vi "历史记录.vi"(9 "动作":enum16{"读取", "添加", "删除", "初始化"}(ring), 11 "历史曲线":cluster{"时间":dbl[], "力":dbl[]}[](array[cluster])) -> (0 "错误输出":errorcluster, 1 "记录大小":i32, 3 "历史曲线":cluster{"时间":dbl[], "力":dbl[]}[](array[cluster]))   [LabVIEW 2015]
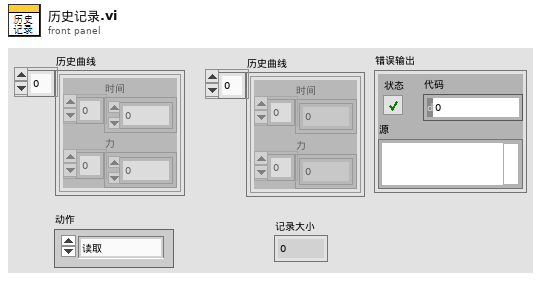
[diagram p1: front panel]
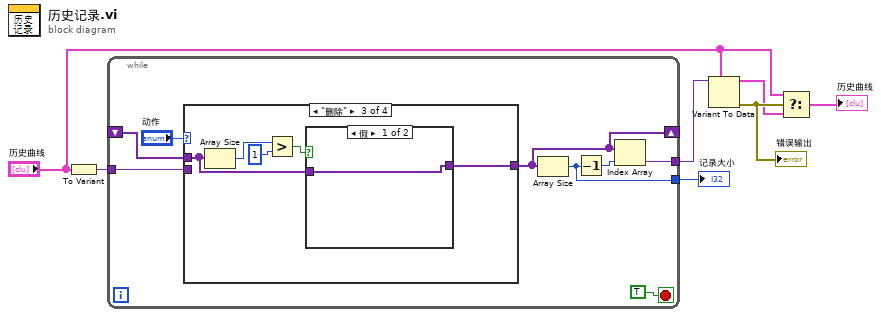
[diagram p0: block diagram]
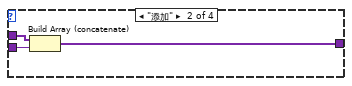
[diagram p3: hidden frame]
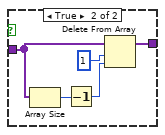
[diagram p4: hidden frame]
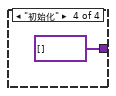
[diagram p5: hidden frame]
diagram:
  n1 = To Variant(anything="历史曲线") -> (Variant=w7:variant)
  n2 = while {
    shift-right: [w8] -> _
    shift-left: _ -> [w13]
    tunnel: w7 -> [w14]
    tunnel: [w11] -> w6
    tunnel: [w9] -> w5
    stop <- TRUE stop-if-true
    n3 = case shown="\"删除\"" "动作" {
      tunnel: w14 -> [_ w18 _ _]
      tunnel: [w16 w17 w24 variant[] []] -> w8
      tunnel: w13 -> [w16 w19 w23 _]
      frame "读取", Default {
      }
      frame "添加" {
        n4 = Build Array (concatenate)(w19, w18) -> (w17:variant[])
      }
      frame "删除" {
        n5 = Array Size(array=w23) -> (size(s)=w22:i32)
        n6 = Greater?(x=w22, y=1) -> (0:w20:bool)
        n7 = case shown="假" w20 {
          tunnel: [w25 w28] -> w24
          tunnel: w23 -> [w25 w26]
          frame False {
          }
          frame True {
            n8 = Array Size(array=w26) -> (size(s)=w29:i32)
            n9 = Decrement(x=w29) -> (x-1=w27:i32)
            n10 = Delete From Array(array=w26, length=1 ("长度"), index=w27) -> (array with subset deleted=w28:variant[])  [unwired: 1 out]
          }
        }
      }
      frame "初始化" {
      }
    }
    n11 = Array Size(array=w8) -> (size(s)=w9:i32)
    n12 = Decrement(x=w9) -> (x-1=w10:i32)
    n13 = Index Array(array=w8, index=w10) -> (element=w11:variant)
  }
  "记录大小" <- w5
  n14 = Variant To Data(type="历史曲线", Variant=w6) -> (data=w3:cluster{"时间":dbl[], "力":dbl[]}[], error out=w4:errorcluster)  [unwired: 1 in]
  "错误输出" <- w4
  n15 = Select(t="历史曲线", s=w4, f=w3) -> (s? t:f=→"历史曲线":cluster{"时间":dbl[], "力":dbl[]}[])
